vi "Sense Holding of Buttons.vi"(0 "Number of Required Repetitions":i32, 2 "Desired Output":bool, 3 "Input":bool) -> (7 "Result":bool)   [LabVIEW 2018]
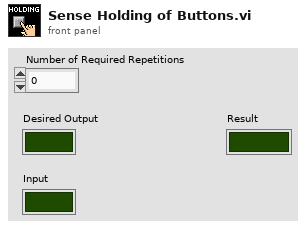
[diagram p1: front panel]
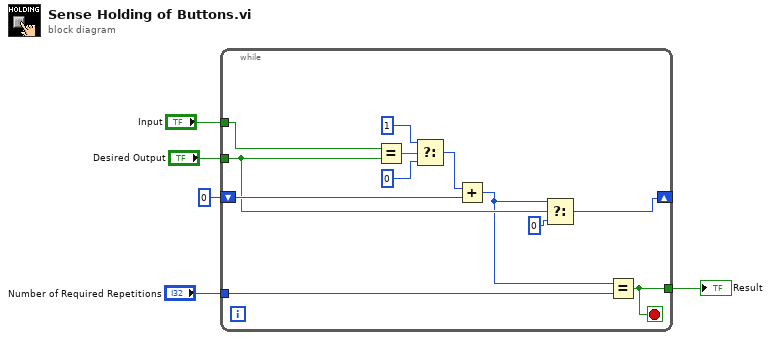
[diagram p0: block diagram]
diagram:
  n1 = while {
    shift-right: [w8] -> _
    shift-left: 0 -> [w12]
    tunnel: "Input" -> [w17]
    tunnel: "Desired Output" -> [w9]
    tunnel: "Number of Required Repetitions" -> [w11]
    tunnel: [w10] -> w1
    stop <- w10 stop-if-true
    n2 = Equal?(x=w17, y=w9) -> (x = y?=w16:bool)
    n3 = Select(t=1, s=w16, f=0) -> (s? t:f=w13:i32)
    n4 = Add(x=w13, y=w12) -> (x+y=w7:i32)
    n5 = Select(t=w7, s=w9, f=0) -> (s? t:f=w8:i32)
    n6 = Equal?(x=w7, y=w11) -> (x = y?=w10:bool)
  }
  "Result" <- w1
